vi "GetListOfPackagesInCEPMFeed.vi"(8 "Error In":errorcluster) -> (0 "Error Out":errorcluster, 3 "Relative Package Paths":path[](array[path]))   [LabVIEW 2019, in "CEPM.lvlib"]
uses:
  CEPM.lvlib
  <vilib>/National Instruments/NIPM API (Beta)/NIPM_API.lvlib
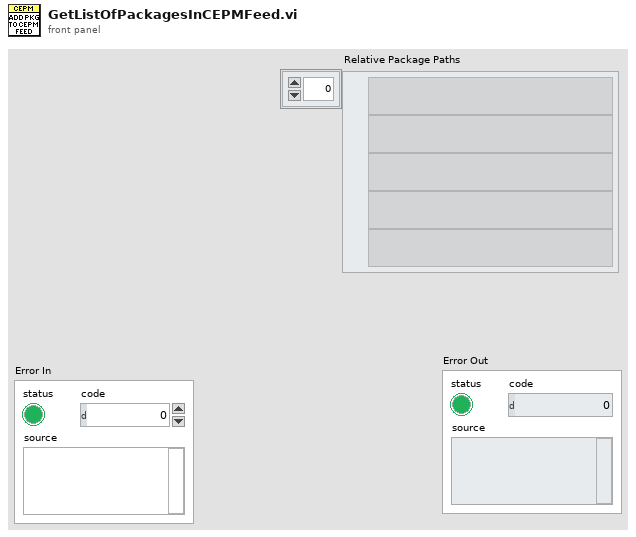
[diagram p1: front panel]
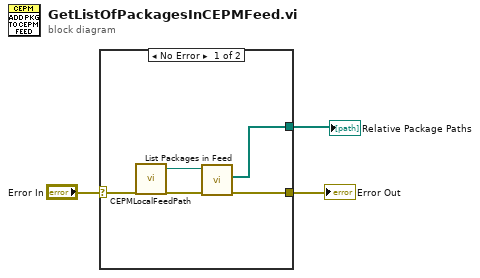
[diagram p0: block diagram]
diagram:
  n1 = case shown="No Error" "Error In" {
    selector: "Error In" -> [w8 w9]
    tunnel: [w5 w9] -> w2
    tunnel: [w4 _] -> w1
    frame No Error {
      n2 = call "CEPMLocalFeedPath.vi"("Error In"=w8) -> ("Error Out"=w6:errorcluster, "CEPM Local Feed Path"=w7:path)  [unwired: 9 in]
      n3 = call <vilib>:"List Packages in Feed.vi"("error in"=w6, "feed folderpath in"=w7) -> ("error out"=w5:errorcluster, "package relative filepaths"=w4:path[])  [unwired: 6 in, 2 out]
    }
    frame Error {
    }
  }
  "Error Out" <- w2
  "Relative Package Paths" <- w1
